vi "Configure Output Relay.vi"(7 "Output Relay Polarity (0: Normal)":u16(ring) items=["Normal", "Reverse"], 8 "error in (no error)":errorcluster, 9 "Enable Polarity Reversal (F: Disable)":bool, 10 "Enable Relay Lock (F: Disable)":bool, 11 "VISA resource name":refnum<visa-resource-name>) -> (0 "error out":errorcluster, 3 "VISA resource name out":refnum<visa-resource-name>)   [LabVIEW 2021, in "Agilent N6900 N7900 Series.lvlib"]
doc: "Locks the output relay and sets its polarity to either normal or reversed. \n\nNote: \n- The values that are set are persistant through a reset. Thus, it may be wise to always set this VI to the desired values.\n- This VI is not valid for N6900 models."
uses:
  <instrlib>/Agilent N6900 N7900 Series/Agilent N6900 N7900 Series.lvlib
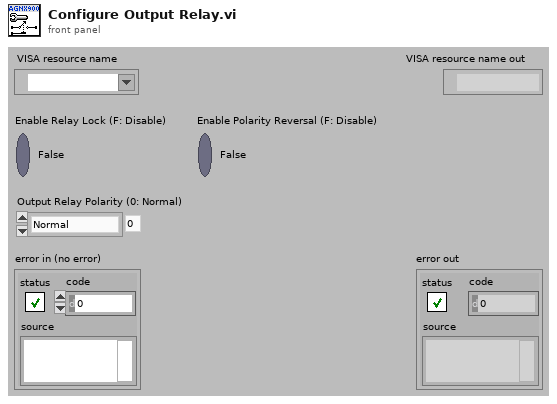
[diagram p1: front panel]
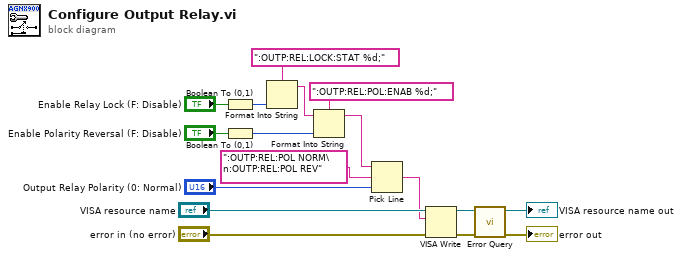
[diagram p0: block diagram]
diagram:
  n1 = Boolean To (0,1)(Boolean="Enable Relay Lock (F: Disable)") -> (0, 1=w2:i16)
  n2 = Boolean To (0,1)(Boolean="Enable Polarity Reversal (F: Disable)") -> (0, 1=w6:i16)
  n3 = Format Into String(format string=":OUTP:REL:LOCK:STAT %d;", w2) -> (resulting string=w4:string)  [unwired: 2 in, 1 out]
  n4 = Format Into String(format string=":OUTP:REL:POL:ENAB %d;", initial string=w4, w6) -> (resulting string=w8:string)  [unwired: 1 in, 1 out]
  n5 = Pick Line(string ("")=w8, multi-line string=":OUTP:REL:POL NORM\n:OUTP:REL:POL REV", line index="Output Relay Polarity (0: Normal)") -> (output string=w9:string)
  n6 = VISA Write(VISA resource name="VISA resource name", write buffer=w9, error in (no error)="error in (no error)") -> (VISA resource name out=w14:refnum<visa-resource-name>, error out=w15:errorcluster)  [unwired: 1 out]
  n7 = call <instrlib>:"Error Query.vi"("error in (no error)"=w15, "VISA resource name"=w14) -> ("error out"=→"error out":errorcluster, "VISA resource name out"=→"VISA resource name out":refnum<visa-resource-name>)  [unwired: 6 in, 2 out]
